vi "Find Target.vi"(8 "error in (no error)":errorcluster, 10 "Name":string="Controller", 11 "SysDef in":refnum<k24>) -> (0 "error out":errorcluster, 2 "Target":refnum<k24>, 3 "SysDef out":refnum<k24>)   [LabVIEW 2020, in "VeriStand SLSC Scripting.lvlib"]
uses:
  VeriStand SLSC Scripting.lvlib
  NationalInstruments.VeriStand.SystemDefinitionAPI
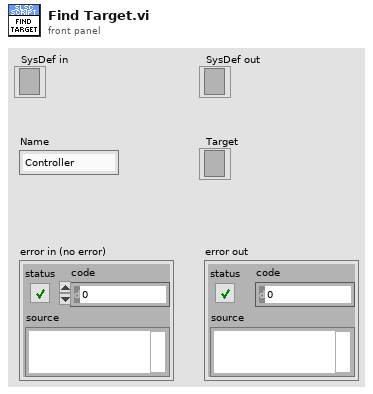
[diagram p1: front panel]
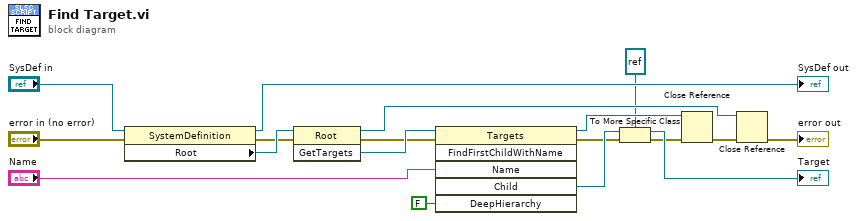
[diagram p0: block diagram]
diagram:
  n1 = property class="SystemDefinition"(reference="SysDef in", error in="error in (no error)") -> (reference out=→"SysDef out":refnum<k24>, error out=w11:errorcluster, "Root"=w15:refnum<k24>)
  n2 = invoke class="Root" method="GetTargets"(reference=w15, error in=w11) -> (reference out=w8:refnum<k24>, error out=w16:errorcluster, "GetTargets"=w17:refnum<k24>)  [unwired: 1 in]
  n3 = invoke class="Targets" method="FindFirstChildWithName"(reference=w17, error in=w16, "Name"="Name", "DeepHierarchy"=FALSE) -> (reference out=w10:refnum<k24>, error out=w3:errorcluster, "Child"=w6:refnum<k24>)  [unwired: 2 in, 3 out]
  n4 = To More Specific Class(target class=refnum<k24> refnum ("reference out"), reference=w6, error in=w3) -> (specific class reference=→"Target":refnum<k24>, error out=w2:errorcluster)
  n5 = Close Reference(reference=w10, error in (no error)=w2) -> (error out=w9:errorcluster)
  n6 = Close Reference(reference=w8, error in (no error)=w9) -> (error out=→"error out":errorcluster)
